vi "init.vi"(0 "EXC3Test in":refnum<class "EXC3Test.lvclass">, 1 "Tolerance":dbl[unit], 5 "Log":refnum<class "ITestLog.lvclass">, 7 "DAQ Channel To Read":refnum<k21>, 9 "Expected Value":dbl[unit], 11 "error in (no error)":errorcluster, 12 "Samples To Read":dbl) -> (4 "EXC3Test out":refnum<class "EXC3Test.lvclass">, 15 "error out":errorcluster)   [LabVIEW 2015, in "EXC3Test.lvclass"]
uses:
  EXC3Test.lvclass
  Model/TestLog/ITestLog/ITestLog.lvclass
  EXC3Test.lvclass/EXC3Test.ctl
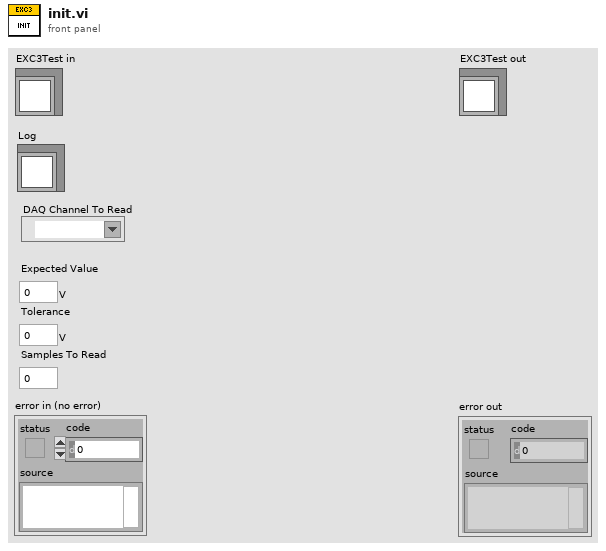
[diagram p1: front panel]
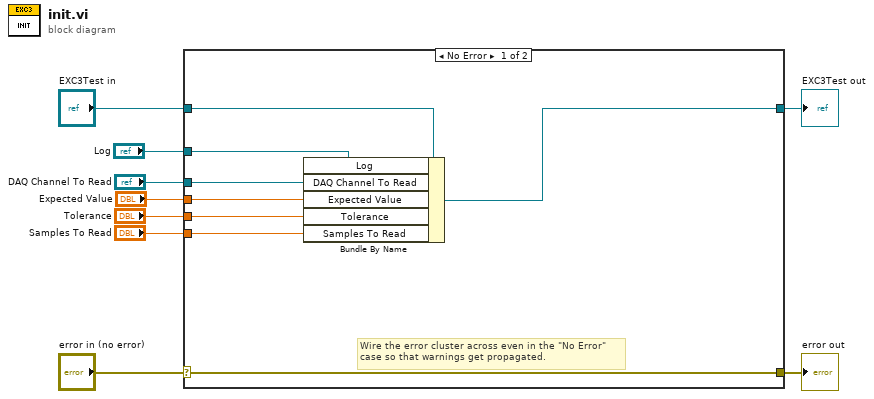
[diagram p0: block diagram]
diagram:
  n1 = case shown="No Error" "error in (no error)" {
    selector: "error in (no error)" -> [w17 w19]
    tunnel: [w17 w19] -> w8
    tunnel: [w15 w18] -> w6
    tunnel: "EXC3Test in" -> [w16 w18]
    tunnel: "Log" -> [w14 _]
    tunnel: "DAQ Channel To Read" -> [w13 _]
    tunnel: "Expected Value" -> [w12 _]
    tunnel: "Tolerance" -> [w11 _]
    tunnel: "Samples To Read" -> [w10 _]
    frame No Error {
      # "Wire the error cluster across even in the \"No Error\"\ncase so that warnings get propagated."
      n2 = Bundle By Name(cluster=w16, "Log"=w14, "DAQ Channel To Read"=w13, "Expected Value"=w12, "Tolerance"=w11, "Samples To Read"=w10) -> (w15:refnum<class "EXC3Test.lvclass">)
    }
    frame Error {
    }
  }
  "error out" <- w8
  "EXC3Test out" <- w6
